vi "PH_Cam_BaseClass.draw CoG.vi"(0 "Image In":T1, 1 "X Resolution":i32, 2 "Y Resolution":i32, 3 "Scale Factor":dbl, 4 "Background Offset":dbl, 5 "error in (no error)":errorcluster, 9 "Color":u32(colorbox)=1985280) -> (14 "Image Out":T1, 19 "error out":errorcluster)   [LabVIEW 2014, in "PH_Cam_BaseClass.lvlib"]
doc: "This VI overlays the center of gravity to an image. It also counts for the fact that the background (mean value) is subtracted."
uses:
  PH_Cam_BaseClass.lvlib
  <vilib>/vision/Image Controls.llb/IMAQ Image.ctl
  <vilib>/vision/NI_Vision_Development_Module.lvlib
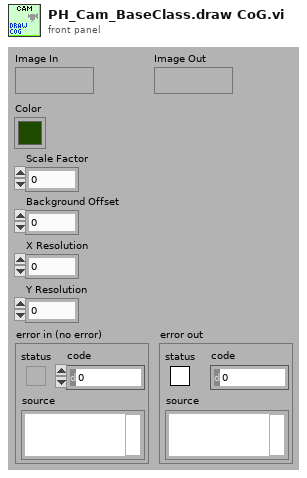
[diagram p1: front panel]
types:
  T1 = typedef "IMAQ Image.ctl" = refnum<image>
  T2 = cluster{"Left":i32, "Top":i32, "Right":i32, "Bottom":i32}
  T3 = cluster{"histogram":u32[], "Minimal Value":sgl, "Maximal Value":sgl, "Starting Value":sgl, "Interval Width":sgl, "Mean Value":sgl, "Standard  Variation":sgl, "Area (pixels)":i32}
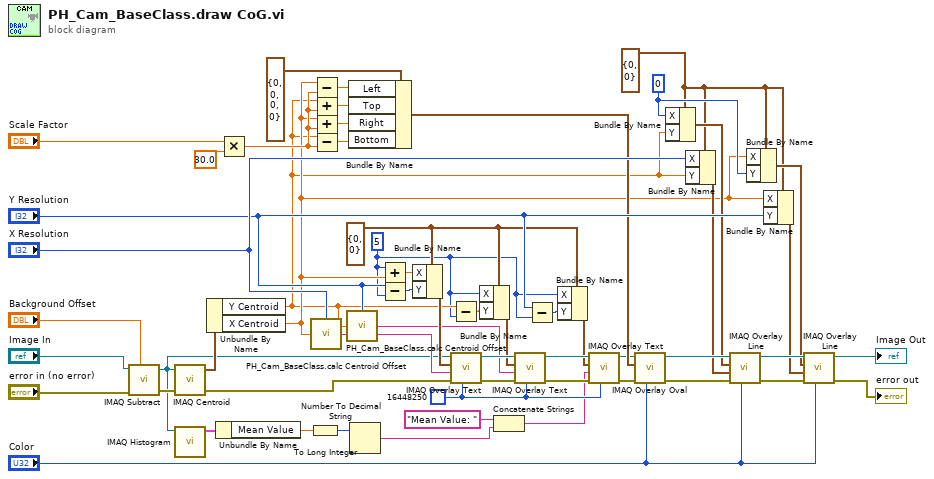
[diagram p0: block diagram]
diagram:
  w4 = cluster{"X":i32, "Y":i32} {"X"=0, "Y"=0} ("Start Point")
  w17 = u32 16448250 ("Color")
  w2 = 5 ("x")
  w36 = 0 ("X")
  w5 = cluster{"X":i32, "Y":i32} {"X"=0, "Y"=0} ("Start Point")
  n1 = call "IMAQ Subtract"("Image Src A"="Image In", "Constant"="Background Offset", "error in (no error)"="error in (no error)") -> ("Image Dst Out"=w1:T1, "error out"=w24:errorcluster)  [unwired: 4 in]
  n2 = call "IMAQ Centroid"("error in (no error)"=w24, "Image"=w1) -> ("error out"=w35:errorcluster, "Centroid"=w34:cluster{"X Centroid":sgl, "Y Centroid":sgl})  [unwired: 2 in]
  n3 = call "IMAQ Histogram"("Image"=w1) -> ("Histogram Report"=w23:T3)  [unwired: 9 in, 1 out]
  n4 = Unbundle By Name(w34) -> ("Y Centroid"=w3:sgl, "X Centroid"=w8:sgl)
  n5 = Unbundle By Name(w23) -> ("Mean Value"=w22:sgl)
  n6 = Multiply(x="Scale Factor", y=30.0) -> (x*y=w49:dbl)
  n7 = To Long Integer(number=w22) -> (32bit integer=w12:i32)
  n8 = call "PH_Cam_BaseClass.calc Centroid Offset.vi"("Resolution"="X Resolution", "Centroid"=w8) -> ("Offset"=w7:string)  [unwired: 13 in]
  n9 = Subtract(x=w8, y=w49) -> (x-y=w33:dbl)
  n10 = Add(x=w3, y=w49) -> (x+y=w32:dbl)
  n11 = Add(x=w8, y=w49) -> (x+y=w31:dbl)
  n12 = Subtract(x=w3, y=w49) -> (x-y=w30:dbl)
  n13 = call "PH_Cam_BaseClass.calc Centroid Offset.vi"("Resolution"="Y Resolution", "Centroid"=w3) -> ("Offset"=w6:string)  [unwired: 13 in]
  n14 = Bundle By Name(cluster=T2 {"Left"=0, "Top"=0, "Right"=0, "Bottom"=0} ("Bounding Rectangle"), "Left"=w33, "Top"=w32, "Right"=w31, "Bottom"=w30) -> (w45:T2)
  n15 = Number To Decimal String(number=w12) -> (decimal integer string=w14:string)  [unwired: 1 in]
  n16 = Add(x=w2, y=w8) -> (x+y=w25:sgl)
  n17 = Subtract(x="Y Resolution", y=w2) -> (x-y=w11:i32)
  n18 = Bundle By Name(cluster=w4, "X"=w25, "Y"=w11) -> (w29:cluster{"X":i32, "Y":i32})
  n19 = Subtract(x=w3, y=w2) -> (x-y=w10:sgl)
  n20 = call "IMAQ Overlay Text"("Text Color (black)"=w17, "error in (no error)"=w35, "String"=w7, "Origin"=w29, "Image"=w1) -> ("error out"=w27:errorcluster, "Image Out"=w28:T1)  [unwired: 5 in]
  n21 = Bundle By Name(cluster=w4, "X"=w2, "Y"=w10) -> (w26:cluster{"X":i32, "Y":i32})
  n22 = Concatenate Strings("Mean Value: " ("string"), w14) -> (w13:string)
  n23 = call "IMAQ Overlay Text"("Text Color (black)"=w17, "error in (no error)"=w27, "String"=w6, "Origin"=w26, "Image"=w28) -> ("error out"=w19:errorcluster, "Image Out"=w21:T1)  [unwired: 5 in]
  n24 = Subtract(x="Y Resolution", y=w2) -> (x-y=w9:i32)
  n25 = Bundle By Name(cluster=w4, "X"=w2, "Y"=w9) -> (w16:cluster{"X":i32, "Y":i32})
  n26 = call "IMAQ Overlay Text"("Text Color (black)"=w17, "error in (no error)"=w19, "String"=w13, "Origin"=w16, "Image"=w21) -> ("error out"=w18:errorcluster, "Image Out"=w20:T1)  [unwired: 5 in]
  n27 = call "IMAQ Overlay Oval"("Color"="Color", "error in (no error)"=w18, "Bounding Rectangle"=w45, "Image"=w20) -> ("error out"=w43:errorcluster, "Image Out"=w41:T1)  [unwired: 6 in]
  n28 = Bundle By Name(cluster=w5, "X"=w36, "Y"=w3) -> (w39:cluster{"X":i32, "Y":i32})
  n29 = Bundle By Name(cluster=w5, "X"="X Resolution", "Y"=w3) -> (w40:cluster{"X":i32, "Y":i32})
  n30 = call "IMAQ Overlay Line"("Color"="Color", "error in (no error)"=w43, "End Point"=w40, "Start Point"=w39, "Image"=w41) -> ("error out"=w44:errorcluster, "Image Out"=w42:T1)  [unwired: 5 in]
  n31 = Bundle By Name(cluster=w5, "X"=w8, "Y"=w36) -> (w38:cluster{"X":i32, "Y":i32})
  n32 = Bundle By Name(cluster=w5, "X"=w8, "Y"="Y Resolution") -> (w37:cluster{"X":i32, "Y":i32})
  n33 = call "IMAQ Overlay Line"("Color"="Color", "error in (no error)"=w44, "End Point"=w37, "Start Point"=w38, "Image"=w42) -> ("error out"=→"error out":errorcluster, "Image Out"=→"Image Out":T1)  [unwired: 5 in]
